vi "UpdateDAQLinescanDisplay.vi"(0 "LinescanSampling":T1 {"MacrotimeCycle" format="%.2f"; "OverflowConstant" format="%.2f"; "BinningMicroS" format="%.2f"}, 1 "MCS Trace":refnum<vi>, 2 "operation":enum16{"initialize", "update"}(ring), 3 "Display Settings":refnum<vi>, 4 "Image Settings":refnum<vi>) -> ()   [LabVIEW 2009]
uses:
  DisplaySettings.ctt
  ImageSettings.ctt
  ScannedImage.ctl
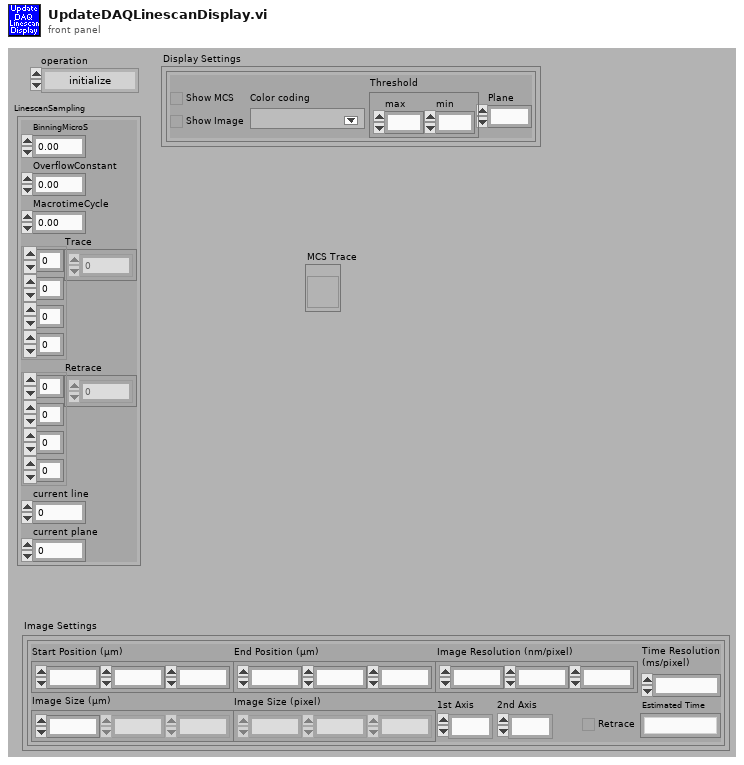
[diagram p1: front panel]
types:
  T1 = typedef "ScannedImage.ctl" = cluster{"BinningMicroS":dbl, "OverflowConstant":dbl, "MacrotimeCycle":dbl, "Trace":u32[][][][], "Retrace":u32[][][][], "current line":i32, "current plane":i32}
  T2 = cluster{"MCS trace":u32[][], "MCS retrace":u32[][], "Image trace":u32[][], "Image retrace":u32[][]}
  T3 = typedef "FIFOSettings.ctt" = cluster{"Measurement":cluster{"Binning (ms)":sgl, "External Trigger Condition":u16, "Stop Condition:":u16, "Stop Count":dbl, "Buffer Size (Photons)":u32, "No of Channels":u16, "Ext Latch Delay":i16}, "ADC":cluster{"Binning (HH)":i16, "Dither Range":i16, "Count Increment":i16, "Mode":u16}, "SYNC":cluster{"SYNC ZC Level (mV)":sgl, "SYNC Freq Divider":u16, "SYNC Holdoff (ps)":sgl, "SYNC Threshold (mV)":sgl}, "TAC":cluster{"TAC Range (ns)":sgl, "TAC Gain":i16, "TAC Offset (%)":sgl, "TAC Limit Low (%)":sgl, "TAC Limit High (%)":sgl}, "Ch 2":cluster{"Ch2 ZC Level (mV)":sgl, "Ch2 Holdoff (ps)":sgl, "Ch2 Threshold (mV)":sgl}, "Ch 3":cluster{"Ch3 ZC Level (mV)":sgl, "Ch3 Holdoff (ps)":sgl, "Ch3 Threshold (mV)":sgl}, "Ch 4":cluster{"Ch4 ZC Level (mV)":sgl, "Ch4 Holdoff (ps)":sgl, "Ch4 Threshold (mV)":sgl}, "Ch1":cluster{"Ch1 ZC Level (mV)":sgl, "Ch1 Holdoff (ps)":sgl, "Ch1 Threshold (mV)":sgl}}
  T4 = cluster{"Start Position (µm)":cluster{"x":dbl, "y":dbl, "z":dbl}, "End Position (µm)":cluster{"x":dbl, "y":dbl, "z":dbl}, "Image Resolution (nm/pixel)":cluster{"x":dbl, "y":dbl, "z":dbl}, "Image Size (µm)":cluster{"x":dbl, "y":dbl, "z":dbl}, "Image Size (pixel)":cluster{"x":u32, "y":u32, "z":u32}, "Time Resolution\n(ms/pixel)":dbl, "1st Axis":u16, "2nd Axis":u16, "Retrace":bool, "Estimated Time":string}
  T5 = typedef "DisplaySettings.ctt" = cluster{"Show MCS":bool, "Show Image":bool, "Color coding":u16, "Plane":u32, "Threshold":cluster{"max":u32, "min":u32}}
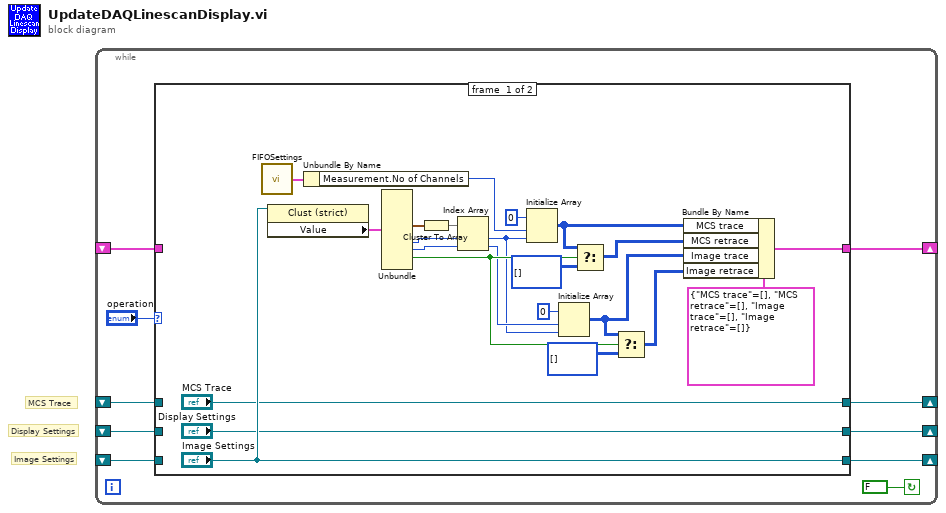
[diagram p0: block diagram]
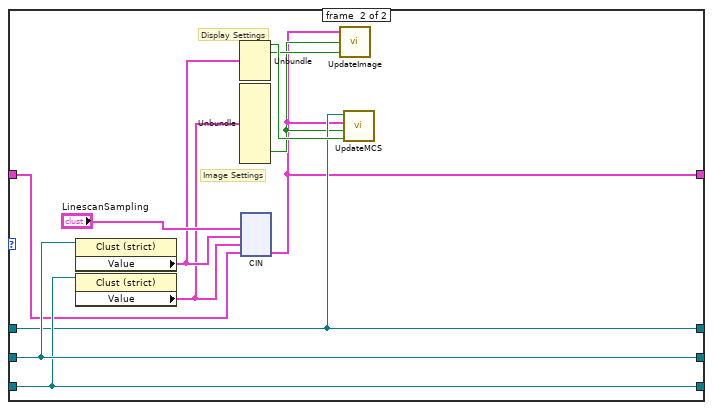
[diagram p2: hidden frame]
diagram:
  # "Image Settings"
  # "Display Settings"
  # "MCS Trace"
  n1 = while {
    shift-right: [w10] -> _
    shift-left: _ -> [w9]
    shift-right: [w7] -> _
    shift-left: _ -> [w6]
    shift-right: [w5] -> _
    shift-left: _ -> [w4]
    shift-right: [w3] -> _
    shift-left: _ -> [w2]
    stop <- FALSE continue-if-true
    n2 = case shown="\"update\"" "operation" {
      tunnel: ["Display Settings" w44] -> w10
      tunnel: w9 -> [_ w44]
      tunnel: ["Image Settings" w43] -> w7
      tunnel: w6 -> [_ w43]
      tunnel: ["MCS Trace" w37] -> w5
      tunnel: w4 -> [_ w37]
      tunnel: [w15 w34] -> w3
      tunnel: w2 -> [_ w41]
      frame #0 {
        n3 = call "FIFOSettings.vi"() -> ("FIFO Settings(out)"=w27:T3)  [unwired: 2 in]
        n4 = property class="Clust (strict)"(reference="Image Settings") -> ("Value"=w32:T4)  [unwired: 1 in, 2 out]
        n5 = Unbundle By Name(w27) -> ("Measurement.No of Channels"=w26:u16)
        n6 = Unbundle(w32) -> ("Image Size (pixel)"=w30:cluster{"x":u32, "y":u32, "z":u32}, "1st Axis"=w28:u16, "2nd Axis"=w20:u16, "Retrace"=w19:bool)  [unwired: 6 out]
        n7 = Cluster To Array(cluster=w30) -> (array=w29:u32[])
        n8 = Index Array(array=w29, index #1=w28, index #2=w20) -> (element #1=w11:u32, element #2=w12:u32)
        n9 = Initialize Array(u32 0 ("element"), w26, w11) -> (w23:u32[][])
        n10 = Initialize Array(u32 0 ("element"), w12, w11) -> (w17:u32[][])
        n11 = Select(t=w23, s=w19, f=u32[][] [] ("initialized array")) -> (s? t:f=w22:u32[][])
        n12 = Select(t=w17, s=w19, f=u32[][] [] ("initialized array")) -> (s? t:f=w16:u32[][])
        n13 = Bundle By Name(cluster=T2 {"MCS trace"=[], "MCS retrace"=[], "Image trace"=[], "Image retrace"=[]}, "MCS trace"=w23, "MCS retrace"=w22, "Image trace"=w17, "Image retrace"=w16) -> (w15:T2)
      }
      frame #1 {
        # "Image Settings"
        # "Display Settings"
        n14 = property class="Clust (strict)"(reference=w44) -> ("Value"=w40:T5)  [unwired: 1 in, 2 out]
        n15 = property class="Clust (strict)"(reference=w43) -> ("Value"=w38:T4)  [unwired: 1 in, 2 out]
        n16 = Unbundle(w40) -> ("Show MCS"=w39:bool, "Show Image"=w36:bool)  [unwired: 3 out]
        n17 = Unbundle(w38) -> ("Retrace"=w35:bool)  [unwired: 9 out]
        n18 = cin("LinescanSampling", w40, w38, w41) -> (w34:T2)  [unwired: 3 in]
        n19 = call "UpdateImage.vi"("Show Image"=w36, "Retrace"=w35, "Update Data"=w34) -> ()
        n20 = call "UpdateMCS.vi"("Show MCS"=w39, "Retrace"=w35, "Update Data"=w34, "MCS Trace"=w37) -> ()
      }
    }
  }
